vi "CSV Player With PtByPt Reporting.vi"() -> ()   [LabVIEW 2011]
uses:
  Controls/Silver Sequence State.ctl
  Controls/Silver Sequence Time.ctl
  Controls/Top Level Control.ctl
  <vilib>/NI/AMC/Message Queue.ctl
  <vilib>/NI/AMC/Message.ctl
  <vilib>/NI/Tools/Keyed Array/KeyedArray.ctl
  Controls/ListBox Test Record.ctl
  Controls/DVR of CSV Tests Data.ctl
  Controls/CSVs Tests Data.ctl
  Controls/Test Column Data.ctl
  Controls/Options DVR.ctl
  Controls/Options.ctl
  Controls/DPL Request.ctl
  Controls/Test Data Record.ctl
  <vilib>/NI/AMC/Read Termination Message.vi
  <vilib>/NI/AMC/Create Single Message.vi
  <vilib>/NI/AMC/Update Message Routing Info.vi
  <vilib>/NI/AMC/Globals.vi
  <userlib>/_OpenG.lib/array/array.llb/Delete Elements from 1D Array (String)__ogtk.vi
  <vilib>/NI/AMC/Send Message.vi
  <vilib>/NI/Tools/Keyed Array/Tools_KeyedArray.lvlib
  <vilib>/NI/AMC/AMC.lvlib
panel:
  in  "Failures":i32(listbox)=-1
  out "Graph":dbl[][](graph)
  in  "Test Signal Selection":u16(ring) items=["<Test Not Completed>"]
  out "Sequence Time":T1 format="%<%H:%M:%S%3u>t"
  out "Sequence State":T2
  in  "Tests":i32[](listbox)
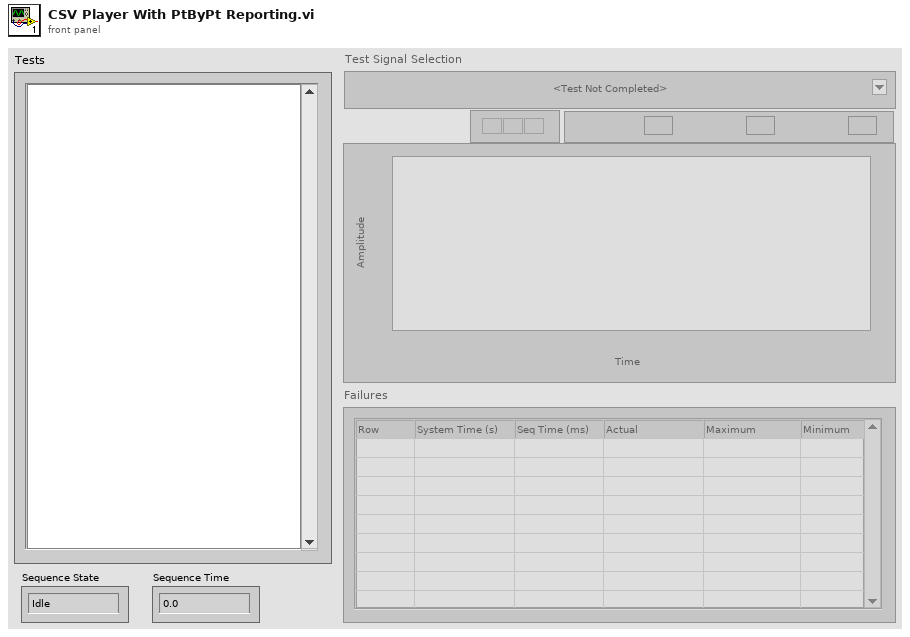
[diagram p1: front panel]
types:
  T1 = typedef "Silver Sequence Time.ctl" = dbl
  T2 = typedef "Silver Sequence State.ctl" = enum16{"Idle", "Running", "SingleStepping", "Paused", "Stopped"}
  T3 = typedef "Top Level Control.ctl" = cluster{"ToGUI":T4, "ToStim":T4, "ToDPL":T4, "RTM":refnum<k9>, "SelectedItems":i32[], "SeqState":refnum<vi>, "SeqTime":refnum<vi>, "ListBox":refnum<vi>, "ListboxTests":T5, "Running?":bool, "#LBoxTests":i32, "RunningTests":T5, "Sel.ItemNames":string[], "TestsData":T6[], "NewTestIdx":i32[], "MsgVal":string, "TopLevel":refnum<vi>, "FP Ref":refnum<vi>, "AppKind":enum32{"invalid app kind", "Development System", "Run Time System", "Student Edition", "Embedded LabVIEW", "Evaluation", "Custom"}, "MuliLB":refnum<vi>, "Ring":refnum<vi>, "Graph":refnum<vi>, "Sel.Signal":string, "DraggedItems":string[], "Colors":u32[], "Options":T7, "ConfiFile":path, "TempCSVs":path[], "RunningCSV":path, "StoppedCSV":path, "DVRToLoad":T6}
  T4 = typedef "AMC.lvlib/Message Queue.ctl" = refnum<queue>
  T5 = typedef "ListBox Test Record.ctl" = cluster{"CSVs":path[], "Filenames":string[]}
  T6 = typedef "DVR of CSV Tests Data.ctl" = refnum<data-value>
  T7 = typedef "Options DVR.ctl" = refnum<data-value>
  T8 = typedef "DPL Request.ctl" = cluster{"TestRec":T6, "Signal":string}
  T9 = typedef "Test Data Record.ctl" = cluster{"Graph Data":dbl[][], "MuliLB Data":string[][]}
  T10 = enum8{"Enabled", "Disabled", "Disabled and Grayed Out"}
  T11 = cluster{"data name":string, "drag data":variant}[]
  T12 = typedef "Excel Refs.ctl" = cluster{"App":refnum<k7>, "Workbooks":refnum<k7>, "Workbook":refnum<k7>, "Sheets":refnum<k7>, "Worksheets":refnum<k7>[], "WorksheetsNames":string[]}
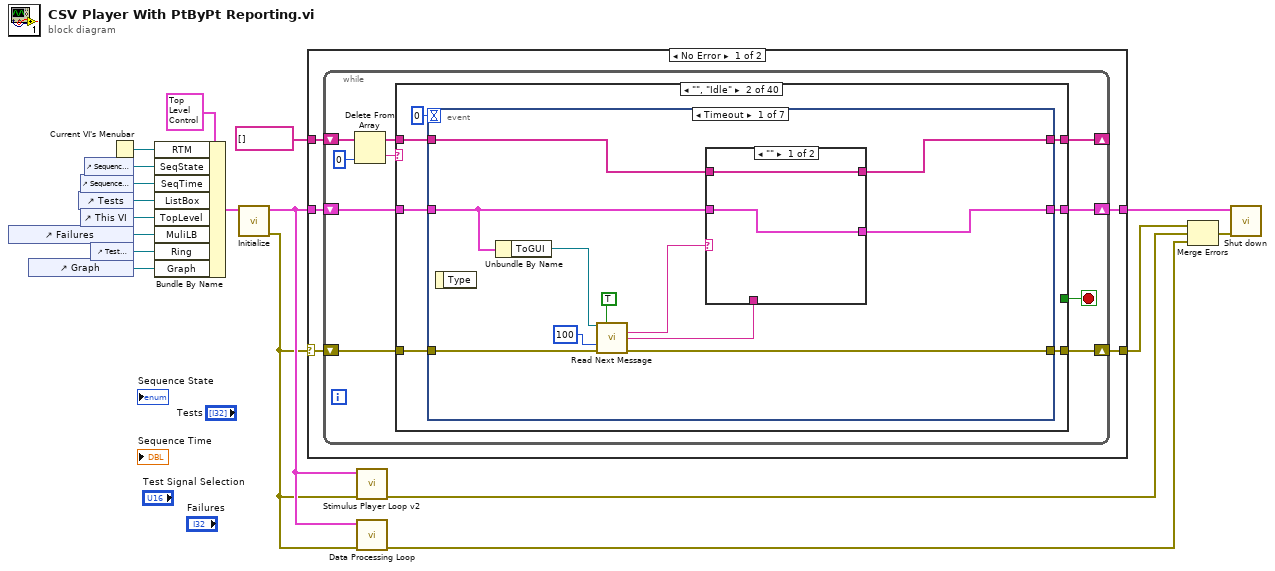
[diagram p0: block diagram]
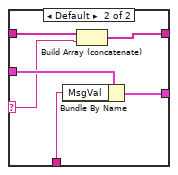
[diagram p3: hidden frame]
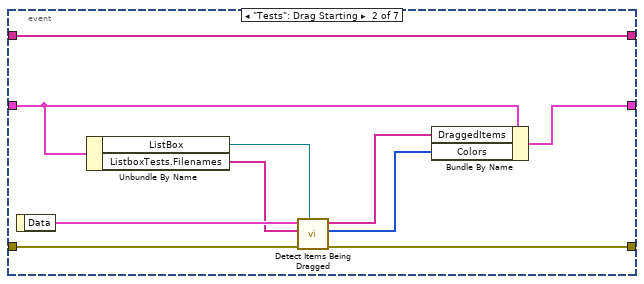
[diagram p4: hidden frame]
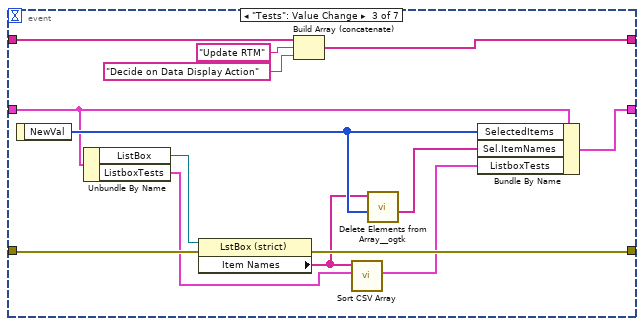
[diagram p5: hidden frame]
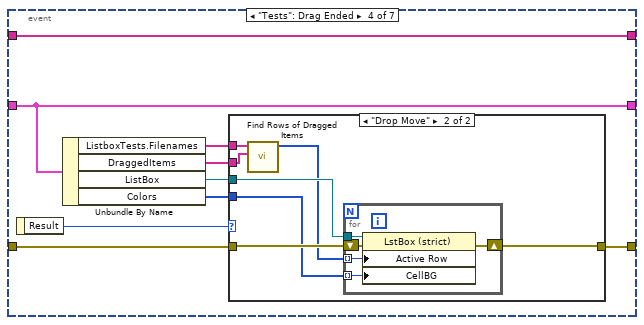
[diagram p6: hidden frame]
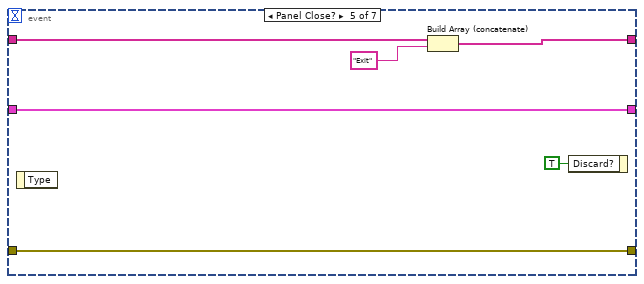
[diagram p8: hidden frame]
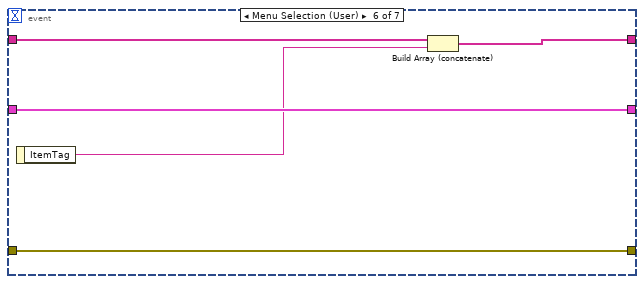
[diagram p9: hidden frame]
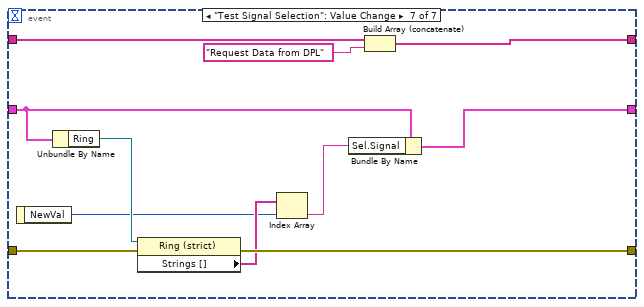
[diagram p10: hidden frame]
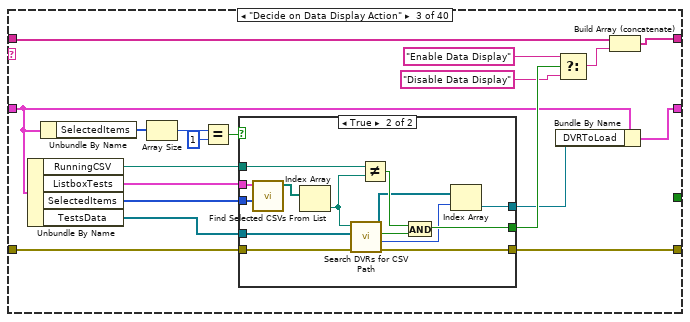
[diagram p11: hidden frame]
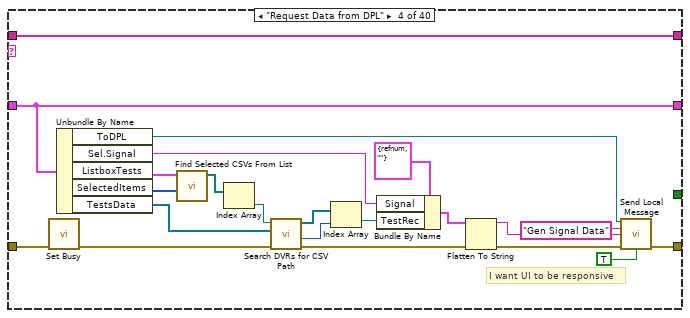
[diagram p13: hidden frame]
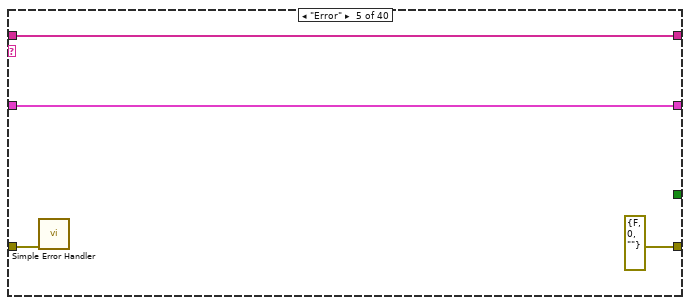
[diagram p14: hidden frame]
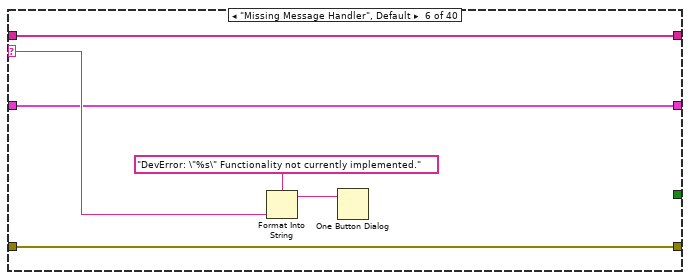
[diagram p15: hidden frame]
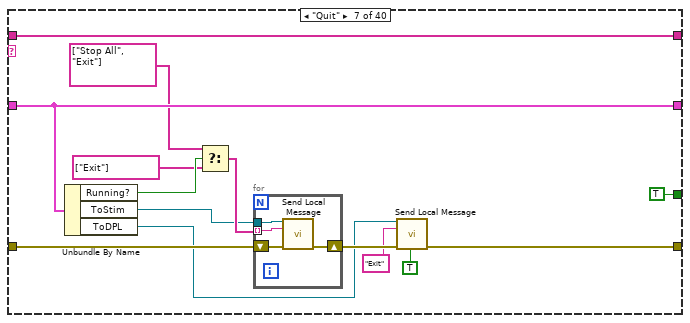
[diagram p16: hidden frame]
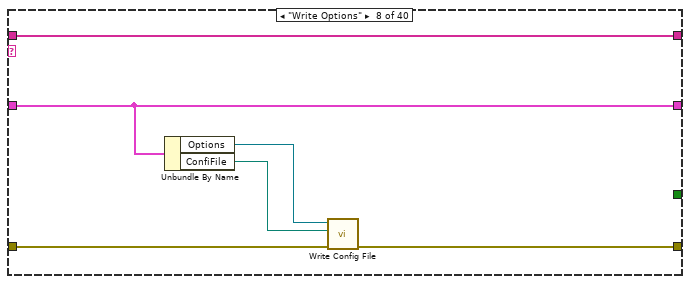
[diagram p17: hidden frame]
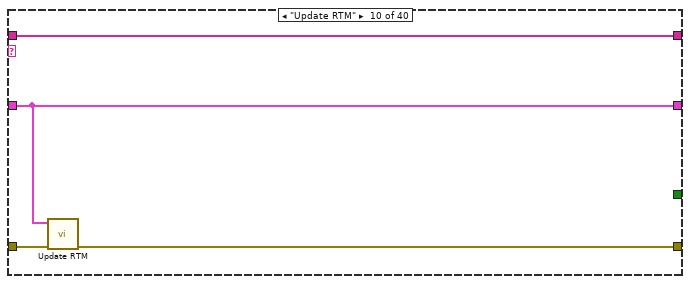
[diagram p19: hidden frame]
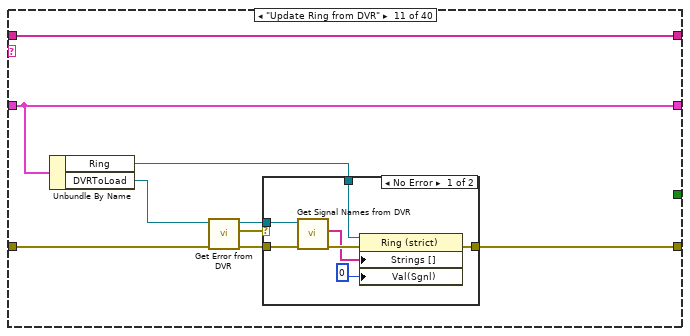
[diagram p20: hidden frame]
diagram:
  n1 = control-ref of="Failures"() -> (w3:refnum<vi>)
  n2 = control-ref of="Graph"() -> (w1:refnum<vi>)
  n3 = control-ref of="Tests"() -> (w7:refnum<vi>)
  n4 = control-ref of="Sequence Time"() -> (w8:refnum<vi>)
  n5 = control-ref of="This VI"() -> (w4:refnum<vi>)
  n6 = control-ref of="Sequence State"() -> (w9:refnum<vi>)
  n7 = control-ref of="Test Signal Selection"() -> (w2:refnum<vi>)
  n8 = Current VI's Menubar() -> (w17:refnum<k9>)
  n9 = Bundle By Name(cluster=T3 {"ToGUI"=refnum, "ToStim"=refnum, "ToDPL"=refnum, "RTM"=refnum, "SelectedItems"=[], "SeqState"=refnum, "SeqTime"=refnum, "ListBox"=refnum, "ListboxTests"={"CSVs"=[], "Filenames"=[]}, "Running?"=FALSE, "#LBoxTests"=0, "RunningTests"={"CSVs"=[], "Filenames"=[]}, "Sel.ItemNames"=[], "TestsData"=[], "NewTestIdx"=[], "MsgVal"="", "TopLevel"=refnum, "FP Ref"=refnum, "AppKind"=enum."invalid app kind", "MuliLB"=refnum, "Ring"=refnum, "Graph"=refnum, "Sel.Signal"="", "DraggedItems"=[], "Colors"=[], "Options"=refnum, "ConfiFile"=path "", "TempCSVs"=[], "RunningCSV"=path "", "StoppedCSV"=path "", "DVRToLoad"=refnum} ("GUI In"), "RTM"=w17, "SeqState"=w9, "SeqTime"=w8, "ListBox"=w7, "TopLevel"=w4, "MuliLB"=w3, "Ring"=w2, "Graph"=w1) -> (w16:T3)
  n10 = call "Initialize.vi"("TopLevel In"=w16) -> ("Error Out"=w5:errorcluster, "TopLevel Out"=w6:T3)  [unwired: 9 in]
  n11 = case shown="No Error" w5 {
    selector: w5 -> [w19 w602]
    tunnel: [w23 w601] -> w15
    tunnel: [w22 w602] -> w14
    tunnel: string[] [] -> [w21 _]
    tunnel: w6 -> [w20 w601]
    frame No Error {
      n12 = while {
        shift-right: [w31] -> w23
        shift-left: w20 -> [w32]
        shift-right: [w26] -> w22
        shift-left: w19 -> [w33]
        shift-right: [w27] -> _
        shift-left: w21 -> [w30]
        stop <- w25 stop-if-true
        n13 = Delete From Array(array=w30, index=0) -> (deleted portion=w24:string, array with subset deleted=w28:string[])  [unwired: 1 in]
        n14 = case shown="\"\", \"Idle\"" w24 {
          selector: w24 -> [_ _ _ _ _ w195 _ _ _ _ _ _ _ _ _ _ _ _ _ _ _ _ _ _ _ _ _ _ _ _ _ _ _ _ _ _ _ _ _ _]
          tunnel: w33 -> [w34 w43 w141 w168 w188 w192 w208 w220 w222 w226 w230 w248 w259 w284 w293 w294 w315 w333 w340 w355 w365 w373 w382 w427 w452 w469 w476 w482 w490 w501 w509 w515 w538 w548 w561 w575 w582 w585 w590 w598]
          tunnel: w32 -> [w36 w42 w133 w186 w191 w193 w209 w218 w224 w227 w236 w251 w255 w282 w291 w299 w321 w332 w344 w359 w367 w371 w377 w424 w449 w466 w477 w483 w489 w503 w507 w517 w529 w545 w559 w574 w583 w587 w592 w599]
          tunnel: [w36 w41 w132 w186 w191 w193 w209 w218 w224 w227 w236 w251 w254 w282 w287 w309 w321 w332 w344 w359 w367 w370 w376 w418 w448 w465 w477 w483 w489 w503 w507 w517 w534 w544 w558 w573 w583 w587 w592 w599] -> w31
          tunnel: w28 -> [w35 w40 w147 w187 w190 w194 w211 w221 w223 w228 w237 w252 w262 w285 w290 w312 w322 w334 w345 w360 w366 w369 w379 w426 w455 w472 w478 w484 w486 w502 w510 w516 w531 w552 w567 w576 w584 w586 w591 w600]
          tunnel: [w35 w38 w146 w187 w190 w194 w211 w221 w223 w228 w237 w252 w262 w285 w289 w311 w322 w334 w336 w351 w366 w368 w378 w425 w445 w462 w478 w484 w485 w502 w505 w516 w537 w551 w566 w571 w584 w586 w589 w600] -> w27
          tunnel: [w34 w39 w140 w173 errorcluster {"status"=FALSE, "code"=0, "source"=""} ("error out") w192 w199 w219 w222 w225 w234 w249 w260 w283 w292 w313 w318 w323 w338 w353 w365 w372 w375 w422 w447 w464 w473 w479 w490 w500 w508 w515 w536 w547 w562 w575 w577 w585 w590 w593] -> w26
          tunnel: [_ _ _ _ _ _ TRUE ("Discard?") _ _ _ _ _ _ _ _ _ _ _ _ _ _ _ _ _ _ _ _ _ _ _ _ _ _ _ _ _ _ _ _ _] -> w25
          frame "------Application Operations------" {
          }
          frame "", "Idle" {
            n15 = event shown="[0] Timeout" {
              selector: _ -> [_ _ _ _ _ _ _]
              dyn-events: _ -> [_ _ _ _ _ _ _]
              timeout: 0 -> [_ _ _ _ _ _ _]
              tunnel: w43 -> [w54 w70 w79 w94 w111 w117 w129]
              tunnel: w42 -> [w47 w66 w80 w92 w112 w118 w124]
              tunnel: [w46 w63 w85 w92 w112 w118 w123] -> w41
              tunnel: w40 -> [w50 w72 w86 w95 w113 w119 w130]
              tunnel: [w51 w69 w77 w91 w111 w117 w128] -> w39
              tunnel: [w49 w72 w84 w95 w110 w116 w121] -> w38
              event Timeout {
                n16 = event-data() -> ()  [unwired: 1 in, 1 out]
                n17 = Unbundle By Name(w47) -> ("ToGUI"=w53:T4)
                n18 = call <vilib>:"Read Next Message.vi"("message queue in"=w53, "ignore error on termination message (F)"=TRUE ("Ignore Error on Termination Message (F)"), "timeout (1 ms)"=100 ("timeout (1ms)"), "error in"=w54) -> ("message name"=w44:string, "message value"=w45:string, "error out"=w51:errorcluster)  [unwired: 4 in, 5 out]
                n19 = case shown="\"\"" w44 {
                  selector: w44 -> [_ w57]
                  tunnel: w50 -> [w56 w62]
                  tunnel: [w56 w61] -> w49
                  tunnel: w47 -> [w55 w60]
                  tunnel: [w55 w59] -> w46
                  tunnel: w45 -> [_ w58]
                  frame "" {
                  }
                  frame Default {
                    n20 = Bundle By Name(cluster=w60, "MsgVal"=w58) -> (w59:T3)
                    n21 = Build Array (concatenate)(w62, w57) -> (w61:string[])
                  }
                }
              }
              event "Tests": Drag Starting {
                n22 = event-data() -> ("Data"=w71:T11)  [unwired: 1 in]
                n23 = Unbundle By Name(w66) -> ("ListBox"=w68:refnum<vi>, "ListboxTests.Filenames"=w67:string[])
                n24 = call "Detect Items Being Dragged.vi"("ListBox"=w68, "error in (no error)"=w70, "LB Filenames"=w67, "Data"=w71) -> ("error out"=w69:errorcluster, "Colors"=w64:u32[], "Items Dragged"=w65:string[])  [unwired: 5 in]
                n25 = Bundle By Name(cluster=w66, "DraggedItems"=w65, "Colors"=w64) -> (w63:T3)
              }
              event "Tests": Value Change {
                n26 = event-data() -> ("NewVal"=w82:i32[])  [unwired: 1 in]
                n27 = Unbundle By Name(w80) -> ("ListBox"=w78:refnum<vi>, "ListboxTests"=w74:T5)
                n28 = property class="LstBox (strict)"(reference=w78, error in=w79) -> (error out=w77:errorcluster, "Item Names"=w76:string[])  [unwired: 1 out]
                n29 = Build Array (concatenate)(w86, "Update RTM", "Decide on Data Display Action") -> (w84:string[])
                n30 = call "Sort CSV Array.vi"("ListBox Tests in"=w74, "New ItemNames"=w76) -> ("Sorted ListBox Tests"=w75:T5)  [unwired: 9 in]
                n31 = call-poly <userlib>:"Delete Elements from Array__ogtk.vi"("indices"=w82, "array"=w76) -> ("deleted elements"=w81:string[])  [unwired: 8 in, 1 out]
                n32 = Bundle By Name(cluster=w80, "SelectedItems"=w82, "Sel.ItemNames"=w81, "ListboxTests"=w75) -> (w85:T3)
              }
              event "Tests": Drag Ended {
                n33 = event-data() -> ("Result"=w93:enum16{"Drop Cancel", "Drop Move", "Drop Copy"})  [unwired: 1 in]
                n34 = Unbundle By Name(w92) -> ("ListboxTests.Filenames"=w90:string[], "DraggedItems"=w89:string[], "ListBox"=w88:refnum<vi>, "Colors"=w87:u32[])
                n35 = case shown="\"Drop Move\"" w93 {
                  tunnel: w94 -> [w96 w101]
                  tunnel: [w96 w97] -> w91
                  tunnel: w90 -> [_ w103]
                  tunnel: w89 -> [_ w102]
                  tunnel: w88 -> [_ w100]
                  tunnel: w87 -> [_ w98]
                  frame Default {
                  }
                  frame "Drop Move" {
                    n36 = call "Find Rows of Dragged Items.vi"("Dragged Items"=w102, "ListBox Strings"=w103) -> ("Rows"=w99:i32[])  [unwired: 9 in]
                    n37 = for {
                      tunnel: w100 -> [w107]
                      tunnel: w99 -> [w106] mode=indexing
                      tunnel: w98 -> [w105] mode=indexing
                      shift-right: [w104] -> w97
                      shift-left: w101 -> [w108]
                      n38 = property class="LstBox (strict)"(reference=w107, error in=w108, "Active Row"=w106, "CellBG"=w105) -> (error out=w104:errorcluster)  [unwired: 1 out]
                    }
                  }
                }
              }
              event Panel Close? {
                n39 = event-data() -> ()  [unwired: 1 in, 1 out]
                n40 = Build Array (concatenate)(w113, "Exit") -> (w110:string[])
                n41 = event-data("Discard?"=TRUE) -> ()  [unwired: 1 in, 1 out]
              }
              event Menu Selection (User) {
                n42 = event-data() -> ("ItemTag"=w115:string)  [unwired: 1 in]
                n43 = Build Array (concatenate)(w119, w115) -> (w116:string[])
              }
              event "Test Signal Selection": Value Change {
                n44 = event-data() -> ("NewVal"=w125:u16)  [unwired: 1 in]
                n45 = Unbundle By Name(w124) -> ("Ring"=w127:refnum<vi>)
                n46 = property class="Ring (strict)"(reference=w127, error in=w129) -> (error out=w128:errorcluster, "Strings []"=w126:string[])  [unwired: 1 out]
                n47 = Index Array(array=w126, index=w125) -> (element=w122:string)
                n48 = Bundle By Name(cluster=w124, "Sel.Signal"=w122) -> (w123:T3)
                n49 = Build Array (concatenate)(w130, "Request Data from DPL") -> (w121:string[])
              }
            }
          }
          frame "Decide on Data Display Action" {
            n50 = Unbundle By Name(w133) -> ("RunningCSV"=w134:path, "ListboxTests"=w144:T5, "SelectedItems"=w143:i32[], "TestsData"=w142:T6[])
            n51 = Unbundle By Name(w133) -> ("SelectedItems"=w145:i32[])
            n52 = Array Size(array=w145) -> (size(s)=w149:i32)
            n53 = Equal?(x=w149, y=1) -> (x = y?=w139:bool)
            n54 = case shown="True" w139 {
              selector: w139 -> [w151 _]
              tunnel: w144 -> [_ w165]
              tunnel: w143 -> [_ w163]
              tunnel: w142 -> [_ w162]
              tunnel: w141 -> [w150 w161]
              tunnel: [w150 w160] -> w140
              tunnel: [w151 w156] -> w138
              tunnel: w134 -> [_ w158]
              tunnel: [_ w152] -> w131
              frame False {
              }
              frame True {
                n55 = call "Find Selected CSVs From List.vi"("Sel.ItemNames"=w163, "ListBox Tests"=w165) -> ("Selected CSVs"=w164:path[])  [unwired: 9 in]
                n56 = Index Array(array=w164) -> (element=w157:path)  [unwired: 1 in]
                n57 = call "Search DVRs for CSV Path.vi"("error in (no error)"=w161, "DVRs"=w162, "CsvPath"=w157) -> ("error out"=w160:errorcluster, "Idx"=w153:i32, "Found?"=w159:bool, "DVRs dup"=w154:T6[])  [unwired: 5 in]
                n58 = Not Equal?(x=w158, y=w157) -> (x != y?=w155:bool)
                n59 = And(x=w155, y=w159) -> (x .and. y?=w156:bool)
                n60 = Index Array(array=w154, index=w153) -> (element=w152:T6)
              }
            }
            n61 = Bundle By Name(cluster=w133, "DVRToLoad"=w131) -> (w132:T3)
            n62 = Select(t="Enable Data Display", s=w138, f="Disable Data Display") -> (s? t:f=w135:string)
            n63 = Build Array (concatenate)(w147, w135) -> (w146:string[])
          }
          frame "Request Data from DPL" {
            # "I want UI to be responsive"
            n64 = call <vilib>:"Set Busy.vi"("error in (no error)"=w168) -> ("error out"=w167:errorcluster)  [unwired: 9 in, 1 out]
            n65 = Unbundle By Name(w186) -> ("ToDPL"=w185:T4, "Sel.Signal"=w174:string, "ListboxTests"=w180:T5, "SelectedItems"=w181:i32[], "TestsData"=w179:T6[])
            n66 = call "Find Selected CSVs From List.vi"("Sel.ItemNames"=w181, "ListBox Tests"=w180) -> ("Selected CSVs"=w183:path[])  [unwired: 9 in]
            n67 = Index Array(array=w183) -> (element=w182:path)  [unwired: 1 in]
            n68 = call "Search DVRs for CSV Path.vi"("error in (no error)"=w167, "DVRs"=w179, "CsvPath"=w182) -> ("error out"=w172:errorcluster, "Idx"=w178:i32, "DVRs dup"=w177:T6[])  [unwired: 5 in, 1 out]
            n69 = Index Array(array=w177, index=w178) -> (element=w175:T6)
            n70 = Bundle By Name(cluster=T8 {"TestRec"=refnum, "Signal"=""} ("DPL Request"), "Signal"=w174, "TestRec"=w175) -> (w171:T8)
            n71 = Flatten To String(anything=w171, error in (no error)=w172) -> (data string=w169:string, error out=w170:errorcluster)  [unwired: 2 in, 1 out]
            n72 = call <vilib>:"Send Local Message.vi"("message queue in"=w185, "message name"="Gen Signal Data" ("Message Name"), "message value"=w169, "error in"=w170, "priority message (F)"=TRUE ("Priority Message (F)")) -> ("error out"=w173:errorcluster)  [unwired: 8 in, 2 out]
          }
          frame "Error" {
            n73 = call <vilib>:"Simple Error Handler.vi"("error in (no error)"=w188) -> ()  [unwired: 1 in, 8 out]
          }
          frame "Missing Message Handler", Default {
            n74 = Format Into String(format string="DevError: \"%s\" Functionality not currently implemented." ("message"), w195) -> (resulting string=w196:string)  [unwired: 2 in, 1 out]
            n75 = One Button Dialog(message=w196) -> ()  [unwired: 2 out]
          }
          frame "Quit" {
            n76 = Unbundle By Name(w209) -> ("Running?"=w207:bool, "ToStim"=w203:T4, "ToDPL"=w201:T4)
            n77 = Select(t=string[] ["Stop All", "Exit"], s=w207, f=string[] ["Exit"]) -> (s? t:f=w204:string[])
            n78 = for {
              shift-right: [w214] -> w202
              shift-left: w208 -> [w215]
              tunnel: w204 -> [w213] mode=indexing
              tunnel: w203 -> [w212]
              n79 = call <vilib>:"Send Local Message.vi"("message queue in"=w212, "message name"=w213, "error in"=w215) -> ("error out"=w214:errorcluster)  [unwired: 10 in, 2 out]
            }
            n80 = call <vilib>:"Send Local Message.vi"("message queue in"=w201, "message name"="Exit", "error in"=w202, "priority message (F)"=TRUE ("Priority Message (F)")) -> ("error out"=w199:errorcluster)  [unwired: 9 in, 2 out]
          }
          frame "Write Options" {
            n81 = Unbundle By Name(w218) -> ("Options"=w216:T7, "ConfiFile"=w217:path)
            n82 = call "Write Config File.vi"("error in (no error)"=w220, "ConfigFile"=w217, "Options"=w216) -> ("error out"=w219:errorcluster)  [unwired: 8 in]
          }
          frame "------GUI Updates------" {
          }
          frame "Update RTM" {
            n83 = call "Update RTM.vi"("error in (no error)"=w226, "TopLevel In"=w227) -> ("error out"=w225:errorcluster)  [unwired: 9 in]
          }
          frame "Update Ring from DVR" {
            n84 = Unbundle By Name(w236) -> ("Ring"=w235:refnum<vi>, "DVRToLoad"=w229:T6)
            n85 = call "Get Error from DVR.vi"("error in (no error)"=w230, "Data Value Reference in"=w229) -> ("error out"=w233:errorcluster, "Error Out"=w231:errorcluster, "Data Value Reference out"=w232:T6)  [unwired: 7 in]
            n86 = case shown="No Error" w231 {
              selector: w231 -> [_ w246]
              tunnel: w235 -> [w239 _]
              tunnel: [w240 w245] -> w234
              tunnel: w233 -> [w244 w245]
              tunnel: w232 -> [w243 _]
              frame No Error {
                n87 = call "Get Signal Names from DVR.vi"("error in (no error)"=w244, "Data Value Reference in"=w243) -> ("error out"=w241:errorcluster, "Signal List"=w238:string[])  [unwired: 7 in, 1 out]
                n88 = property class="Ring (strict)"(reference=w239, error in=w241, "Strings []"=w238, "Val(Sgnl)"=u16 0 ("Value (Signaling)")) -> (error out=w240:errorcluster)  [unwired: 1 out]
              }
              frame Error {
                n89 = call <vilib>:"General Error Handler.vi"("error in (no error)"=w246) -> ()  [unwired: 10 in, 5 out]
              }
            }
          }
          frame "Clear Ring" {
            n90 = Unbundle By Name(w251) -> ("Ring"=w247:refnum<vi>)
            n91 = property class="Ring (strict)"(reference=w247, error in=w248, "Strings []"=string[] ["<Test Not Completed>"]) -> (error out=w249:errorcluster)  [unwired: 1 out]
          }
          frame "Set LB Pass/Fail Color" {
            n92 = Unbundle By Name(w255) -> ("TestsData"=w257:T6[], "NewTestIdx"=w256:i32[], "ListBox"=w261:refnum<vi>, "ListboxTests.Filenames"=w258:string[])
            n93 = for {
              tunnel: w261 -> [w272]
              tunnel: w258 -> [w266]
              tunnel: w257 -> [w265]
              shift-right: [w270] -> w260
              shift-left: w259 -> [w267]
              tunnel: w256 -> [w263] mode=indexing
              n94 = Index Array(array=w265, index=w263) -> (element=w264:T6)
              n95 = call "Get Path&PassFail from DVR.vi"("error in (no error)"=w267, "Data Value Reference in"=w264) -> ("error out"=w273:errorcluster, "FileName"=w274:string, "Pass?"=w269:bool)  [unwired: 5 in, 2 out]
              n96 = Search 1D Array(1D array=w266, element=w274) -> (index of element=w271:i32)  [unwired: 1 in]
              n97 = case shown="True" w269 {
                tunnel: [u32 65330 u32 16719872] -> w268
                frame True {
                }
                frame False {
                }
              }
              n98 = property class="LstBox (strict)"(reference=w272, error in=w273, "Active Row"=w271, "CellBG"=w268) -> (error out=w270:errorcluster)  [unwired: 1 out]
            }
            n99 = Bundle By Name(cluster=w255, "NewTestIdx"=i32[] [] ("Pass?ColorIdx")) -> (w254:T3)
          }
          frame "Set Running Tests to Yellow" {
            n100 = Unbundle By Name(w282) -> ("FP Ref"=w278:refnum<vi>, "ListBox"=w281:refnum<vi>, "RunningTests.Filenames"=w280:string[], "ListboxTests.Filenames"=w279:string[])
            n101 = call "Set Running Tests to Color.vi"("Color"=u32 16775978, "FP Ref"=w278, "Error In"=w284, "Listbox Tests"=w279, "Running Tests"=w280, "Tests"=w281) -> ("Error Out"=w283:errorcluster)  [unwired: 5 in]
          }
          frame "Revert All Running Test Colors" {
            # "We have stopped, so if there were any running tests... revert their colors back to previous"
            n102 = call "Revert Running Test Colors.vi"("Error In"=w293, "TopLevel in"=w291, "QSM In"=w290) -> ("Error Out"=w292:errorcluster, "TopLevel out"=w288:T3, "QSM out"=w289:string[])  [unwired: 6 in]
            n103 = Bundle By Name(cluster=w288, "RunningTests"=T5 {"CSVs"=[], "Filenames"=[]}) -> (w287:T3)
          }
          frame "Revert One Running Test Color" {
            # "TODO: Make this less of a mess"
            # "Trick the revert all subVI into just reverting one"
            n104 = Unbundle By Name(w299) -> ("RunningTests.Filenames"=w306:string[], "RunningTests.CSVs"=w307:path[], "StoppedCSV"=w295:path)
            n105 = Search 1D Array(1D array=w307, element=w295) -> (index of element=w305:i32)  [unwired: 1 in]
            n106 = Delete From Array(array=w306, index=w305) -> (deleted portion=w303:string, array with subset deleted=w298:string[])  [unwired: 1 in]
            n107 = Delete From Array(array=w307, index=w305) -> (deleted portion=w302:path, array with subset deleted=w304:path[])  [unwired: 1 in]
            n108 = Build Array(w303) -> (w300:string[])
            n109 = Build Array(w302) -> (w301:path[])
            n110 = Bundle By Name(cluster=w299, "RunningTests.Filenames"=w300, "RunningTests.CSVs"=w301) -> (w308:T3)
            n111 = Empty Array?(array=w298) -> (empty?=w297:bool)
            n112 = Not(x=w297) -> (.not. x?=w296:bool)
            n113 = call "Revert Running Test Colors.vi"("Error In"=w294, "TopLevel in"=w308, "QSM In"=w312) -> ("Error Out"=w313:errorcluster, "TopLevel out"=w310:T3, "QSM out"=w311:string[])  [unwired: 6 in]
            n114 = Bundle By Name(cluster=w310, "Running?"=w296, "RunningTests.Filenames"=w298, "RunningTests.CSVs"=w304) -> (w309:T3)
          }
          frame "Highlight Test Blue" {
            n115 = Unbundle By Name(w321) -> ("ListBox"=w319:refnum<vi>, "ListboxTests.CSVs"=w320:path[], "RunningCSV"=w314:path)
            n116 = Search 1D Array(1D array=w320, element=w314) -> (index of element=w317:i32)  [unwired: 1 in]
            n117 = property class="LstBox (strict)"(reference=w319, error in=w315, "Active Row"=w317, "CellBG"=u32 8971007) -> (error out=w318:errorcluster)  [unwired: 1 out]
          }
          frame "Populate Data Display" {
            n118 = Unbundle By Name(w332) -> ("MuliLB"=w331:refnum<vi>, "MsgVal"=w330:string)
            n119 = Unflatten From String(type=T9 {"Graph Data"=[], "MuliLB Data"=[]} ("Data Record"), binary string=w330, error in (no error)=w333) -> (value=w328:T9, error out=w327:errorcluster)  [unwired: 2 in, 1 out]
            n120 = Unbundle By Name(w328) -> ("Graph Data"=→"Graph":dbl[][], "MuliLB Data"=w325:string[][])
            n121 = property class="MCListbox (strict)"(reference=w331, error in=w327, "ItemNames"=w325) -> (error out=w324:errorcluster)  [unwired: 1 out]
            n122 = call <vilib>:"Unset Busy.vi"("error in (no error)"=w324) -> ("error out"=w323:errorcluster)  [unwired: 10 in]
          }
          frame "Disable Data Display" {
            n123 = Unbundle By Name(w344) -> ("Graph"=w341:refnum<vi>, "Ring"=w342:refnum<vi>, "MuliLB"=w343:refnum<vi>)
            n124 = Build Array(w341, w342, w343) -> (w339:refnum<vi>[])
            n125 = for {
              shift-right: [w347] -> w338
              shift-left: w340 -> [w349]
              tunnel: w339 -> [w348] mode=indexing
              tunnel: T10."Disabled and Grayed Out" ("Disabled") -> [w346]
              n126 = property class="Ctl"(reference=w348, error in=w349, "DisabledEnum"=w346) -> (error out=w347:errorcluster)  [unwired: 1 out]
            }
            n127 = Build Array (concatenate)(w345, "Clear Ring") -> (w336:string[])
          }
          frame "Enable Data Display" {
            n128 = Unbundle By Name(w359) -> ("Graph"=w356:refnum<vi>, "Ring"=w357:refnum<vi>, "MuliLB"=w358:refnum<vi>)
            n129 = Build Array(w356, w357, w358) -> (w354:refnum<vi>[])
            n130 = for {
              shift-right: [w362] -> w353
              shift-left: w355 -> [w364]
              tunnel: w354 -> [w363] mode=indexing
              tunnel: T10."Enabled" ("Disabled") -> [w361]
              n131 = property class="Ctl"(reference=w363, error in=w364, "DisabledEnum"=w361) -> (error out=w362:errorcluster)  [unwired: 1 out]
            }
            n132 = Build Array (concatenate)(w360, "Update Ring from DVR") -> (w351:string[])
          }
          frame "-------Menu Selections-------" {
          }
          frame "Import CSV File(s)..." {
            n133 = call "Import CSV Files.vi"("error in (no error)"=w373, "TopLevel in"=w371, "QSM in"=w369) -> ("error out"=w372:errorcluster, "TopLevel out"=w370:T3, "QSM out"=w368:string[])  [unwired: 6 in]
          }
          frame "Import CSV Worksheets From Excel..." {
            n134 = File Dialog(4:"Excel file containing NIVS tabe based tests" ("pattern label"), 5:"Select Worksheets..." ("button label"), 6:"*.xls;*.xlsx" ("pattern (all files)"), 7:"Select Excel file" ("prompt"), 8:w382) -> (0:w381:errorcluster, 1:w374:bool, 3:w380:path)  [unwired: 2 in, 1 out]
            n135 = case shown="False" w374 {
              tunnel: w381 -> [w404 w414]
              tunnel: w380 -> [w398 _]
              tunnel: w379 -> [w394 w416]
              tunnel: [w393 w416] -> w378
              tunnel: w377 -> [w392 w415]
              tunnel: [w388 w415] -> w376
              tunnel: [w391 w412] -> w375
              frame False {
                n136 = call "Open Excel File.vi"("error in (no error)"=w404, "File"=w398) -> ("error out"=w403:errorcluster, "ExcelRefs"=w402:T12)  [unwired: 8 in]
                n137 = Strip Path(path=w398) -> (stripped path=w390:path)  [unwired: 1 out]
                n138 = call "Select Desired Excel Worksheets.vi"("error in (no error)"=w403, "ExcelRefs in"=w402) -> ("error out"=w400:errorcluster, "Selected Worksheets"=w399:string[], "ExcelRefs dup"=w401:T12)  [unwired: 6 in, 1 out]
                n139 = for {
                  shift-right: [w406] -> w397
                  shift-left: w400 -> [w410]
                  shift-right: [w407] -> w396
                  shift-left: w401 -> [w411]
                  tunnel: w399 -> [w409] mode=indexing
                  tunnel: w390 -> [w408]
                  tunnel: [w405] -> w387 mode=indexing
                  n140 = call "Save Specific Worksheet as CSV.vi"("error in (no error)"=w410, "Destination Directory"=w408, "Worksheet Name"=w409, "ExcelRefs in"=w411) -> ("error out"=w406:errorcluster, "New CSV File"=w405:path, "ExcelRefs dup"=w407:T12)  [unwired: 5 in]
                }
                n141 = call "Close Excel File.vi"("Error In"=w397, "ExcelRefs"=w396) -> ("Error Out"=w395:errorcluster)  [unwired: 9 in]
                n142 = call "Add CSVs to Test List.vi"("error in (no error)"=w395, "Array"=w387, "TopLevel in in"=w392, "QSM in in"=w394) -> ("error out"=w391:errorcluster, "TopLevel in out"=w389:T3, "QSM in out"=w393:string[])  [unwired: 5 in]
                n143 = Bundle By Name(cluster=w389, "TempCSVs"=w387) -> (w388:T3)
              }
              frame True {
                n144 = call "Clear Specific Error.vi"("error in (no error)"=w414, "code"=43) -> ("error out"=w412:errorcluster)  [unwired: 9 in]
              }
            }
          }
          frame "Delete" {
            n145 = Unbundle By Name(w424) -> ("#LBoxTests"=w421:i32)
            n146 = call "Delete.vi"("error in (no error)"=w427, "TopLevel In"=w424, "QSM In"=w426) -> ("error out"=w423:errorcluster, "TopLevel Out"=w418:T3, "QSM Out"=w425:string[])  [unwired: 6 in]
            n147 = Unbundle By Name(w418) -> ("ListBox"=w417:refnum<vi>, "#LBoxTests"=w420:i32)
            n148 = Greater Than 0?(x=w420) -> (x > 0?=w419:bool)
            n149 = case shown="False" w419 {
              tunnel: w423 -> [w431 w440]
              tunnel: [w430 w439] -> w422
              tunnel: w421 -> [w429 w438]
              tunnel: w418 -> [_ w437]
              tunnel: w417 -> [w428 _]
              frame False {
                n150 = for {
                  N: w429 -> [_]
                  shift-right: [w436] -> w430
                  shift-left: w431 -> [w435]
                  tunnel: w428 -> [w434]
                  i -> [w432]
                  n151 = property on="Property Node" class="LstBox (strict)"(reference=w434, error in=w435, "Active Row"=w432, "CellBG"=u32 16777215) -> (error out=w436:errorcluster)  [unwired: 1 out]
                }
              }
              frame True {
                n152 = call "Fix Coloring Offset.vi"("error in (no error)"=w440, "# LB Tests"=w438, "TopLevel"=w437) -> ("error out"=w439:errorcluster)  [unwired: 8 in]
              }
            }
          }
          frame "Run All" {
            n153 = Unbundle By Name(w449) -> ("ToStim"=w454:T4, "ListboxTests.Filenames"=w443:string[], "ListboxTests.CSVs"=w442:path[])
            n154 = Flatten To String(anything=w442, error in (no error)=w452) -> (data string=w450:string, error out=w451:errorcluster)  [unwired: 2 in, 1 out]
            n155 = call <vilib>:"Send Local Message.vi"("message queue in"=w454, "message name"="Play" ("Message Name"), "message value"=w450, "error in"=w451) -> ("error out"=w447:errorcluster)  [unwired: 9 in, 2 out]
            n156 = Build Array (concatenate)(w455, "Update RTM", "Set Running Tests to Yellow") -> (w445:string[])
            n157 = Bundle By Name(cluster=w449, "Running?"=TRUE, "RunningTests.Filenames"=w443, "RunningTests.CSVs"=w442) -> (w448:T3)
          }
          frame "Run Selected" {
            n158 = Unbundle By Name(w466) -> ("ToStim"=w471:T4, "ListboxTests"=w460:T5, "Sel.ItemNames"=w456:string[], "SelectedItems"=w459:i32[])
            n159 = call "Find Selected CSVs From List.vi"("Sel.ItemNames"=w459, "ListBox Tests"=w460) -> ("Selected CSVs"=w458:path[])  [unwired: 9 in]
            n160 = Flatten To String(anything=w458, error in (no error)=w469) -> (data string=w467:string, error out=w468:errorcluster)  [unwired: 2 in, 1 out]
            n161 = call <vilib>:"Send Local Message.vi"("message queue in"=w471, "message name"="Play" ("Message Name"), "message value"=w467, "error in"=w468) -> ("error out"=w464:errorcluster)  [unwired: 9 in, 2 out]
            n162 = Build Array (concatenate)(w472, "Update RTM", "Set Running Tests to Yellow") -> (w462:string[])
            n163 = Bundle By Name(cluster=w466, "Running?"=TRUE, "RunningTests.CSVs"=w458, "RunningTests.Filenames"=w456) -> (w465:T3)
          }
          frame "Stop All" {
            n164 = Unbundle By Name(w477) -> ("ToStim"=w475:T4)
            n165 = call <vilib>:"Send Local Message.vi"("message queue in"=w475, "message name"="Stop All", "error in"=w476) -> ("error out"=w473:errorcluster)  [unwired: 10 in, 2 out]
          }
          frame "Stop Current Test" {
            n166 = Unbundle By Name(w483) -> ("ToStim"=w481:T4)
            n167 = call <vilib>:"Send Local Message.vi"("message queue in"=w481, "message name"="Stop", "error in"=w482) -> ("error out"=w479:errorcluster)  [unwired: 10 in, 2 out]
          }
          frame "Exit" {
            n168 = Unbundle By Name(w489) -> ("Running?"=w488:bool)
            n169 = case shown="True" w488 {
              tunnel: [TRUE ("T button?") w492] -> w487
              frame False {
              }
              frame True {
                n170 = Two Button Dialog(message="Tests are currently running. If you exit now, they will be stopped. Are you sure? ", 1:"No" ("F button name (\"Cancel\")"), 2:"Yes" ("T button name (\"OK\")")) -> (T button?=w492:bool)
              }
            }
            n171 = case shown="True" w487 {
              tunnel: w486 -> [w496 w499]
              tunnel: [w496 w497] -> w485
              frame False {
              }
              frame True {
                n172 = Build Array (concatenate)(w499, "Quit" ("T button name (\"OK\")")) -> (w497:string[])
              }
            }
          }
          frame "About" {
            n173 = call "About.vi"("error in (no error)"=w501) -> ("error IO"=w500:errorcluster)  [unwired: 10 in]
          }
          frame "Options" {
            n174 = Unbundle By Name(w507) -> ("Options"=w506:T7)
            n175 = call "Options.vi"("Error In"=w509, "Options DVR In"=w506) -> ("Error Out"=w508:errorcluster, "Cancelled?"=w504:bool)  [unwired: 8 in]
            n176 = case shown="False" w504 {
              tunnel: w510 -> [w513 w514]
              tunnel: [w512 w514] -> w505
              frame False {
                n177 = Build Array (concatenate)(w513, "Write Options") -> (w512:string[])
              }
              frame True {
              }
            }
          }
          frame "-------Stim Loop Msg Handlers-------" {
          }
          frame "New Test Record" {
            # "Stim loop finished a CSV and is sending results"
            n178 = call "Replace or Append Test Data DVR.vi"("error in (no error)"=w538, "TopLevel Out in"=w529) -> ("error out"=w536:errorcluster, "CsvPath"=w520:path, "TopLevel Out out"=w528:T3)  [unwired: 7 in]
            n179 = Unbundle By Name(w528) -> ("ListboxTests.CSVs"=w525:path[], "SelectedItems"=w527:i32[])
            n180 = Index Array(array=w527) -> (element=w526:i32)  [unwired: 1 in]
            n181 = Index Array(array=w525, index=w526) -> (element=w524:path)
            n182 = Equal?(x=w524, y=w520) -> (x = y?=w523:bool)
            n183 = case shown="True" w523 {
              tunnel: w531 -> [w539 w542]
              tunnel: [w539 w540] -> w530
              frame False {
              }
              frame True {
                n184 = Build Array (concatenate)(w542, "Decide on Data Display Action") -> (w540:string[])
              }
            }
            n185 = Unbundle By Name(w528) -> ("RunningTests"=w535:T5, "RunningCSV"=w519:path)
            n186 = Not Equal?(x=w519, y=w520) -> (x != y?=w522:bool)
            n187 = call "Remove Recieved Test From Running List.vi"("Finished Test"=w520, "Running Tests in"=w535) -> ("Running Tests out"=w533:T5)  [unwired: 9 in]
            n188 = Select(t=w519, s=w522, f=path "") -> (s? t:f=w518:path)
            n189 = Bundle By Name(cluster=w528, "RunningTests"=w533, "RunningCSV"=w518) -> (w534:T3)
            n190 = Build Array (concatenate)(w530, "Set LB Pass/Fail Color") -> (w537:string[])
          }
          frame "Started CSV" {
            n191 = Unbundle By Name(w545) -> ("MsgVal"=w546:string)
            n192 = Unflatten From String(type=path "", binary string=w546, error in (no error)=w548) -> (value=w543:path, error out=w547:errorcluster)  [unwired: 2 in, 1 out]
            n193 = Build Array (concatenate)(w552, "Highlight Test Blue") -> (w551:string[])
            n194 = Bundle By Name(cluster=w545, "RunningCSV"=w543) -> (w544:T3)
          }
          frame "Stopped CSV" {
            # "Stim loop stopped a CSV as requested and is sending which one it was"
            n195 = Unbundle By Name(w559) -> ("RunningCSV"=w555:path, "MsgVal"=w560:string)
            n196 = Unflatten From String(type=path "", binary string=w560, error in (no error)=w561) -> (value=w557:path, error out=w562:errorcluster)  [unwired: 2 in, 1 out]
            n197 = Not Equal?(x=w555, y=w557) -> (x != y?=w556:bool)
            n198 = Select(t=w555, s=w556, f=path "") -> (s? t:f=w554:path)
            n199 = Build Array (concatenate)(w567, "Revert One Running Test Color", "Update RTM") -> (w566:string[])
            n200 = Bundle By Name(cluster=w559, "RunningCSV"=w554, "StoppedCSV"=w557) -> (w558:T3)
          }
          frame "Finished" {
            # "Stim loop has finished its CSV queue either because it played all of them or because it was commanded to stop all"
            n201 = Build Array (concatenate)(w576, "Revert All Running Test Colors", "Update RTM") -> (w571:string[])
            n202 = Bundle By Name(cluster=w574, "Running?"=FALSE, "RunningCSV"=path "") -> (w573:T3)
          }
          frame "Stim Error" {
            n203 = Unbundle By Name(w583) -> ("MsgVal"=w581:string)
            n204 = Unflatten From String(type=errorcluster {"status"=FALSE, "code"=0, "source"=""} ("error constant"), binary string=w581, error in (no error)=w582) -> (value=w578:errorcluster, error out=w579:errorcluster)  [unwired: 2 in, 1 out]
            n205 = Merge Errors(w579, w578) -> (w577:errorcluster)
          }
          frame "-------Data Loop Msg Handlers-------" {
          }
          frame "New Test Data" {
            n206 = Build Array (concatenate)(w591, "Populate Data Display") -> (w589:string[])
          }
          frame "DPL Error" {
            n207 = Unbundle By Name(w599) -> ("MsgVal"=w597:string)
            n208 = Unflatten From String(type=errorcluster {"status"=FALSE, "code"=0, "source"=""} ("error constant"), binary string=w597, error in (no error)=w598) -> (value=w594:errorcluster, error out=w595:errorcluster)  [unwired: 2 in, 1 out]
            n209 = Merge Errors(w595, w594) -> (w593:errorcluster)
          }
        }
      }
    }
    frame Error {
    }
  }
  n210 = call "Stimulus Player Loop v2.vi"("Error In"=w5, "TopLevel"=w6) -> ("Error Out"=w11:errorcluster)  [unwired: 9 in]
  n211 = call "Data Processing Loop.vi"("Error In"=w5, "TopLevel"=w6) -> ("Error Out"=w12:errorcluster)  [unwired: 9 in]
  n212 = Merge Errors(w14, w11, w12) -> (w13:errorcluster)
  n213 = call "Shut down.vi"("Error In"=w13, "GUI"=w15) -> ()  [unwired: 10 in]
